vi "creat_control_channels.vi"(10 "control_string":string[][](array[string])) -> (2 "control_channels":T2(array[cluster]))   [LabVIEW 2024]
panel:
  out "control_channel":T1={"channel_name"="", "on/off"=FALSE, "Line(s)"="Dev1/port0/line0:1"}
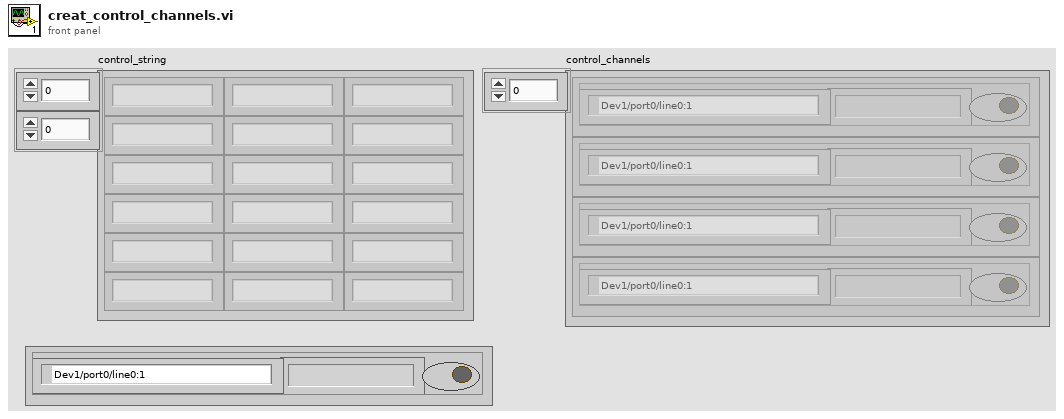
[diagram p1: front panel]
types:
  T1 = cluster{"channel_name":string, "on/off":bool, "Line(s)":tag}
  T2 = cluster{"channel_name":string, "on/off":bool, "Line(s)":tag}[]
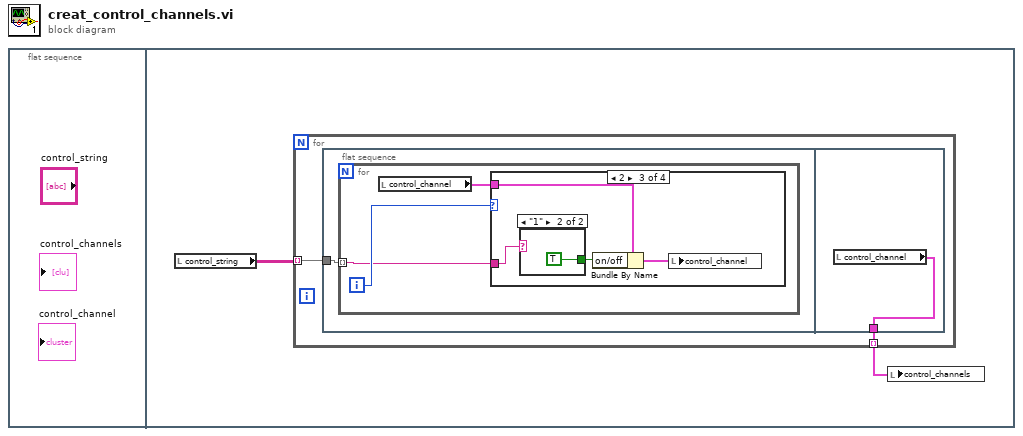
[diagram p0: block diagram]
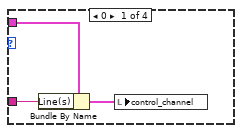
[diagram p2: hidden frame]
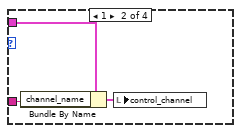
[diagram p3: hidden frame]
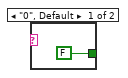
[diagram p4: hidden frame]
diagram:
  n1 = flat-sequence {
    frame #0 {
    }
    frame #1 {
      n2 = local read "control_string"() -> (w2:string[][])
      n3 = for {
        tunnel: w2 -> [w4] mode=indexing
        tunnel: [w3] -> w1 mode=indexing
        n4 = flat-sequence {
          tunnel: w4 -> [w5]
          tunnel: [w21] -> w3
          frame #0 {
            n5 = for {
              tunnel: w5 -> [w6] mode=indexing
              i -> [w8]
              n6 = local read "control_channel"() -> (w7:T1)
              n7 = case shown="2" w8 {
                tunnel: w7 -> [w10 w12 w16 _]
                tunnel: w6 -> [w11 w13 w18 _]
                frame 0 {
                  n8 = Bundle By Name(cluster=w10, "Line(s)"=w11) -> (w9:T1)
                  n9 = local write "control_channel"(w9) -> ()
                }
                frame 1 {
                  n10 = Bundle By Name(cluster=w12, "channel_name"=w13) -> (w14:T1)
                  n11 = local write "control_channel"(w14) -> ()
                }
                frame 2 {
                  n12 = case shown="\"1\"" w18 {
                    tunnel: [FALSE TRUE] -> w15
                    frame "0", Default {
                    }
                    frame "1" {
                    }
                  }
                  n13 = Bundle By Name(cluster=w16, "on/off"=w15) -> (w17:T1)
                  n14 = local write "control_channel"(w17) -> ()
                }
                frame 3, Default {
                }
              }
            }
          }
          frame #1 {
            n15 = local read "control_channel"() -> (w21:T1)
          }
        }
      }
      n16 = local write "control_channels"(w1) -> ()
    }
  }
